vi "Get_Position_Info.vi"(2 "Analysis Info cluster":T1[](array[typedef]) {"Sd Error in Variance" format="%.2f"; "Skew_u" format="%.2f"; "% u'/U" format="%.2f"; "Sd Error in Mean" format="%.2f"; "Kurt_u" format="%.2f"; "u^4" format="%.2f"; "u^3" format="%.2f"; "U" format="%.2f"; "u^2" format="%.2f"}, 3 "Setup file string":string) -> (0 "Analysis Info cluster 2":T1[](array[typedef]) {"Sd Error in Variance" format="%.2f"; "Skew_u" format="%.2f"; "% u'/U" format="%.2f"; "Sd Error in Mean" format="%.2f"; "Kurt_u" format="%.2f"; "u^4" format="%.2f"; "u^3" format="%.2f"; "U" format="%.2f"; "u^2" format="%.2f"})   [LabVIEW 2012]
uses:
  Controls/Analysis_info_cluster.ctl
  Controls/Inst_type.ctl
  Controls/Instrument_Array.ctl
  Controls/Post_Process.ctl
  Controls/User_Specific_mode.ctl
  Globals/Meas_global.vi
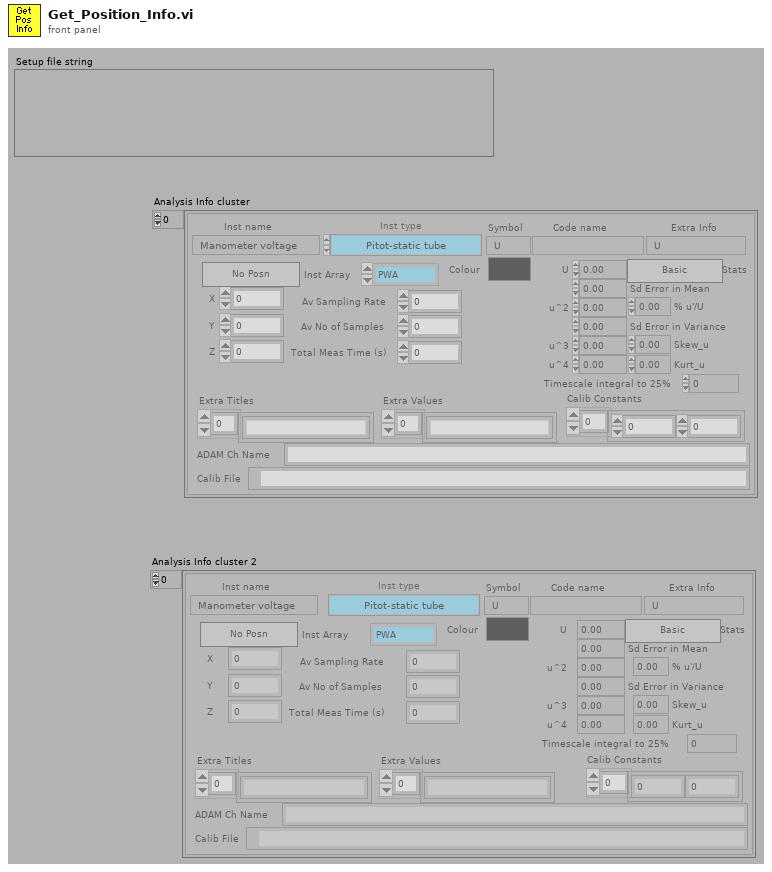
[diagram p1: front panel]
types:
  T1 = typedef "Analysis_info_cluster.ctl" = cluster{"Colour":u32, "Inst type":T2, "Inst name":string, "Symbol":string, "Code name":string, "Extra Info":string, "Inst Array":T3, "Extra Titles":string[], "Extra Values":string[], "U":dbl, "u^2":dbl, "u^3":dbl, "u^4":dbl, "Skew_u":dbl, "Kurt_u":dbl, "Sd Error in Mean":dbl, "% u'/U":dbl, "X":dbl, "Y":dbl, "Z":dbl, "Timescale integral to 25%":dbl, "Sd Error in Variance":dbl, "Calib File":path, "Calib Constants":dbl[], "Output Position":bool, "Full Stats":bool, "Av Sampling Rate":dbl, "Av No of Samples":dbl, "Total Meas Time (s)":dbl, "ADAM Ch Name":string}
  T2 = typedef "Inst_type.ctl" = enum16{"Propeller anemometer", "Raw voltage", "Pressure Transducer", "Pitot-static tube", "Preston tube", "Hot wire", "Cross wire 1", "Cross wire 2", "Generic Linear", "Generic Polynomial", "Generic BackPoly", "Fast FID", "Thermocouple", "Cold wire", "Pulsed Wire", "LDA Vel", "LDA Tran time", "LDA Arr time"}
  T3 = typedef "Instrument_Array.ctl" = enum16{"PWA", "LDA", "Analogue"}
  T4 = typedef "Post_Process.ctl" = enum16{"Take New Data", "Post Process Raw Data File"}
  T5 = typedef "User_Specific_mode.ctl" = enum16{"Check VI only", "Run VI"}
  T6 = cluster{"Values[0]":dbl, "Values[1]":dbl, "Values[2]":dbl}
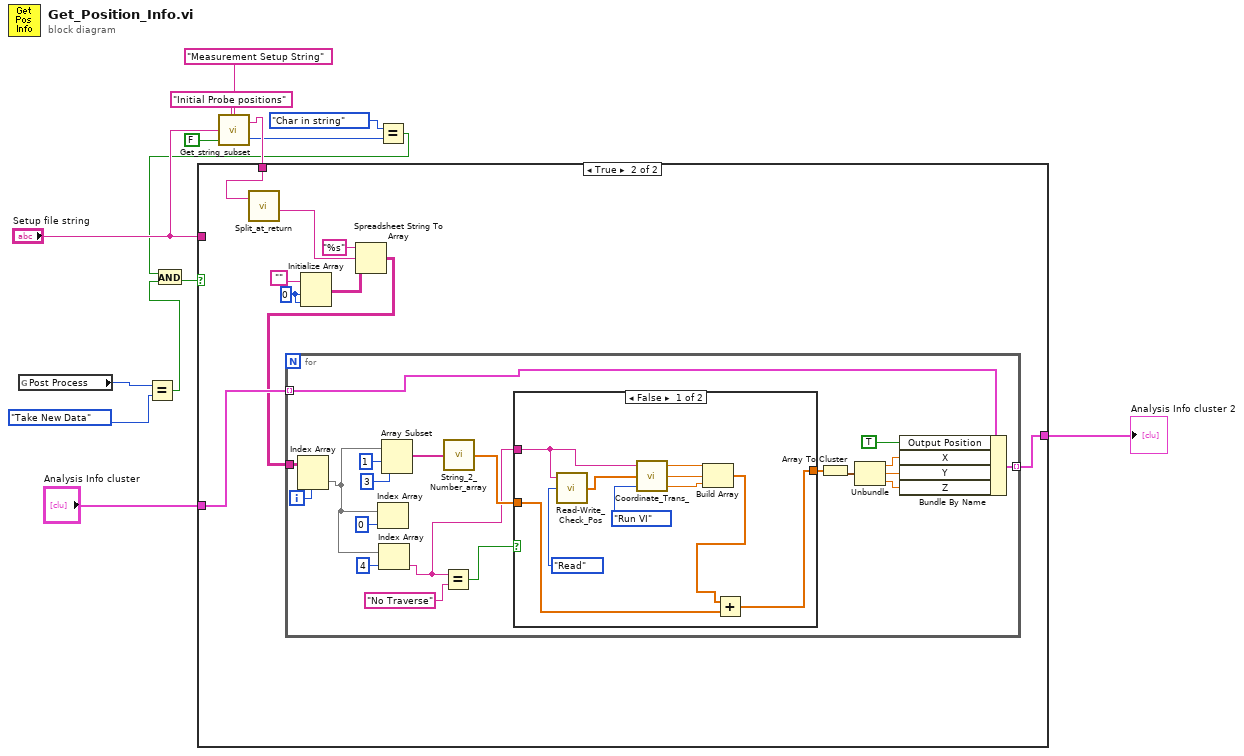
[diagram p0: block diagram]
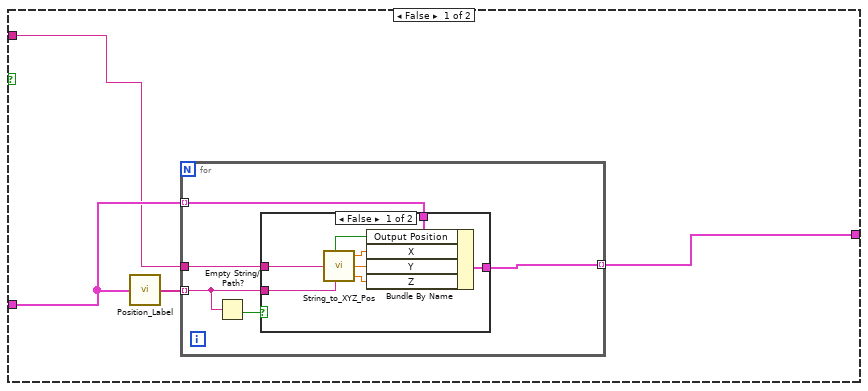
[diagram p2: hidden frame]
diagram:
  n1 = global read "Meas_global.vi" "Post Process"() -> (w14:T4)
  n2 = Equal?(x=w14, y=Post_Process."Take New Data" ("Post Process")) -> (x = y?=w3:bool)
  n3 = call "Get_string_subset.vi"("String Name"="Measurement Setup String", "Show Dialog?"=FALSE, "String to split"="Setup file string", "File Label"="Initial Probe positions") -> ("Status"=w7:enum16{"Char in string", "Char not in string"}, "Output string"=w10:string)
  n4 = Equal?(x=enum16{"Char in string", "Char not in string"}."Char in string" ("Status"), y=w7) -> (x = y?=w6:bool)
  n5 = And(x=w6, y=w3) -> (x .and. y?=w5:bool)
  n6 = case shown="True" w5 {
    tunnel: w10 -> [_ w37]
    tunnel: "Setup file string" -> [w16 _]
    tunnel: "Analysis Info cluster" -> [w18 w35]
    tunnel: [w15 w34] -> w1
    frame False {
      n7 = call "Position_Label.vi"("Analysis Info cluster"=w18) -> ("Position Label"=w17:string[])
      n8 = for {
        tunnel: w18 -> [w22] mode=indexing
        tunnel: [w23] -> w15 mode=indexing
        tunnel: w17 -> [w20] mode=indexing
        tunnel: w16 -> [w21]
        n9 = Empty String/Path?(string/path=w20) -> (empty?=w19:bool)
        n10 = case shown="False" w19 {
          tunnel: [w31 w32] -> w23
          tunnel: w22 -> [w30 w32]
          tunnel: w20 -> [w29 _]
          tunnel: w21 -> [w28 _]
          frame False {
            n11 = call "String_to_XYZ_Pos.vi"("Input string"=w28, "Position label"=w29) -> ("Some labels found"=w24:bool, "X"=w27:dbl, "Y"=w26:dbl, "Z"=w25:dbl)  [unwired: 2 in]
            n12 = Bundle By Name(cluster=w30, "Output Position"=w24, "X"=w27, "Y"=w26, "Z"=w25) -> (w31:T1)
          }
          frame True {
          }
        }
      }
    }
    frame True {
      w40 = 0 ("Dimension Size")
      n13 = call "Split_at_return.vi"("String"=w37) -> ("after substring"=w36:string)  [unwired: 1 in, 3 out]
      n14 = Initialize Array("", w40, w40) -> (w41:string[][])
      n15 = Spreadsheet String To Array(format string="%s", spreadsheet string=w36, array type (2D Dbl)=w41) -> (array=w33:string[][])  [unwired: 1 out]
      n16 = for {
        tunnel: [w49] -> w34 mode=indexing
        tunnel: w35 -> [w46] mode=indexing
        tunnel: w33 -> [w44]
        i -> [w45]
        n17 = Index Array(array=w44, index (row)=w45) -> (element=w43:string[])  [unwired: 1 in]
        n18 = Index Array(array=w43, index=0) -> ()  [unwired: 1 out]
        n19 = Index Array(array=w43, index=4) -> (element=w48:string)
        n20 = Array Subset(array=w43, index=1, length=3) -> (w47:string[])
        n21 = Equal?(x=w48, y="No Traverse" ("x")) -> (x = y?=w58:bool)
        n22 = call "String_2_Number_array.vi"("Input String"=w47) -> ("Values"=w56:dbl[])
        n23 = case shown="False" w58 {
          tunnel: [w70 w72] -> w57
          tunnel: w56 -> [w71 w72]
          tunnel: w48 -> [w64 _]
          frame False {
            n24 = call "Read-Write_Check_Pos.vi"("Mode"=enum16{"Read", "Write"}."Read", "Traverse Name"=w64) -> ("Position Output"=w63:dbl[])  [unwired: 1 in]
            n25 = call "Coordinate_Trans_.vi"("Simulate/Run"=User_Specific_mode."Run VI", "Input Position"=w63, "Traverse Name"=w64) -> ("Z"=w67:dbl, "Y"=w68:dbl, "X"=w69:dbl)
            n26 = Build Array(w69, w68, w67) -> (w66:dbl[])
            n27 = Add(x=w66, y=w71) -> (x+y=w70:dbl[])
          }
          frame True {
          }
        }
        n28 = Array To Cluster(array=w57) -> (cluster=w55:T6)
        n29 = Unbundle(w55) -> ("Values[0]"=w54:dbl, "Values[1]"=w53:dbl, "Values[2]"=w52:dbl)
        n30 = Bundle By Name(cluster=w46, "Output Position"=TRUE, "X"=w54, "Y"=w53, "Z"=w52) -> (w49:T1)
      }
    }
  }
  "Analysis Info cluster 2" <- w1
